vi "DAQ_Test.vi"() -> ()   [LabVIEW 2011]
uses:
  range_ni6009_TypDef.ctl
  OnOffTypeDef.ctl
panel:
  out "Array":variant[](array[variant])
  out "data 2":waveform(dbl)[](graph)
  in  "ChannelEnable":T1[](array[typedef])
  in  "range (V) 2":T2=enum."10"
  in  "Enable":bool
  in  "Channel (0.1.2.3)":string="0"
  in  "range (V)":T2=enum."10"
  in  "Range":T2[](array[typedef])
  out "Counter":i32
  out "OK":bool
  in  "timeout":dbl=1.0
  in  "Trigger":bool
  out "error out":errorcluster
  out "x-y":u32(graph)
  out "data":waveform(dbl)[](graph)
  in  "stop":bool
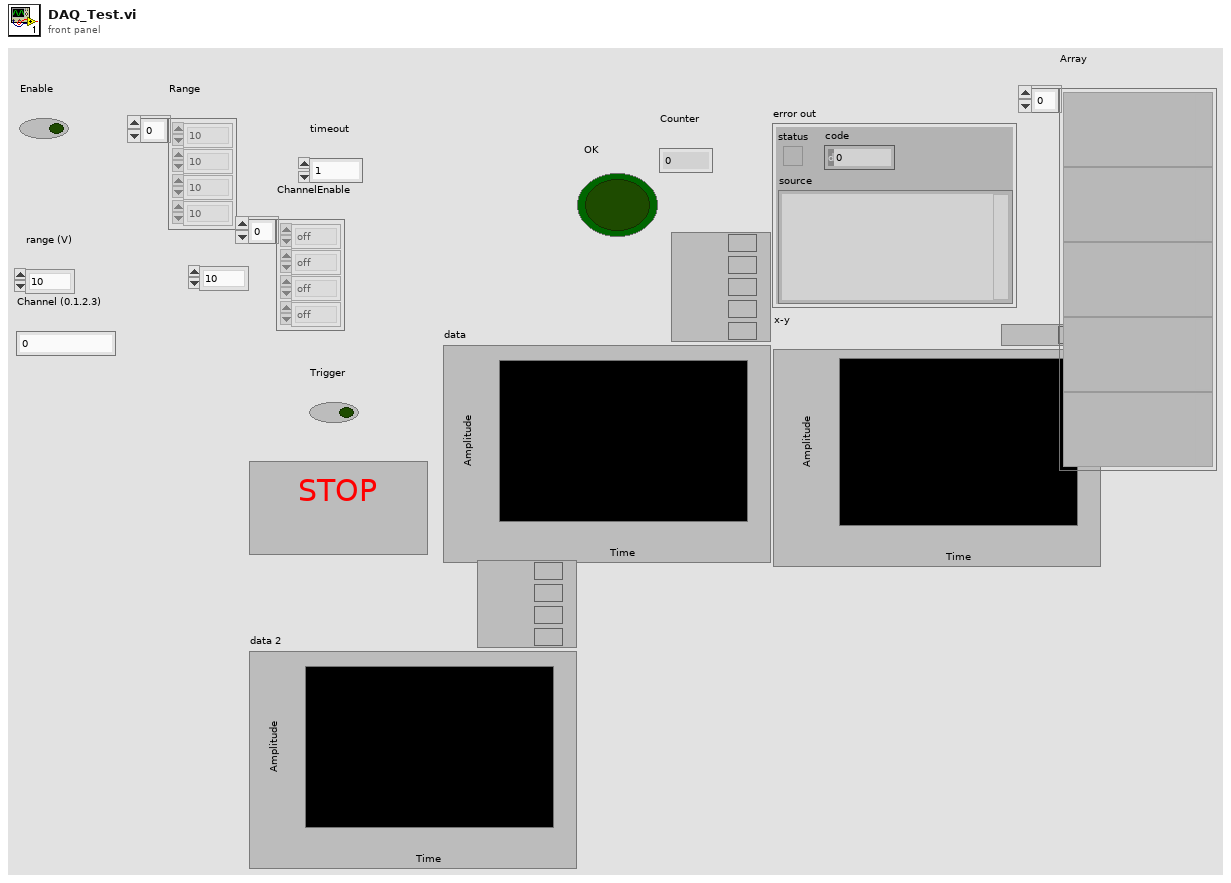
[diagram p1: front panel]
types:
  T1 = typedef "OnOffTypeDef.ctl" = enum16{"off", "on"}
  T2 = typedef "range_ni6009_TypDef.ctl" = enum16{"1", "2", "4", "5", "10"}
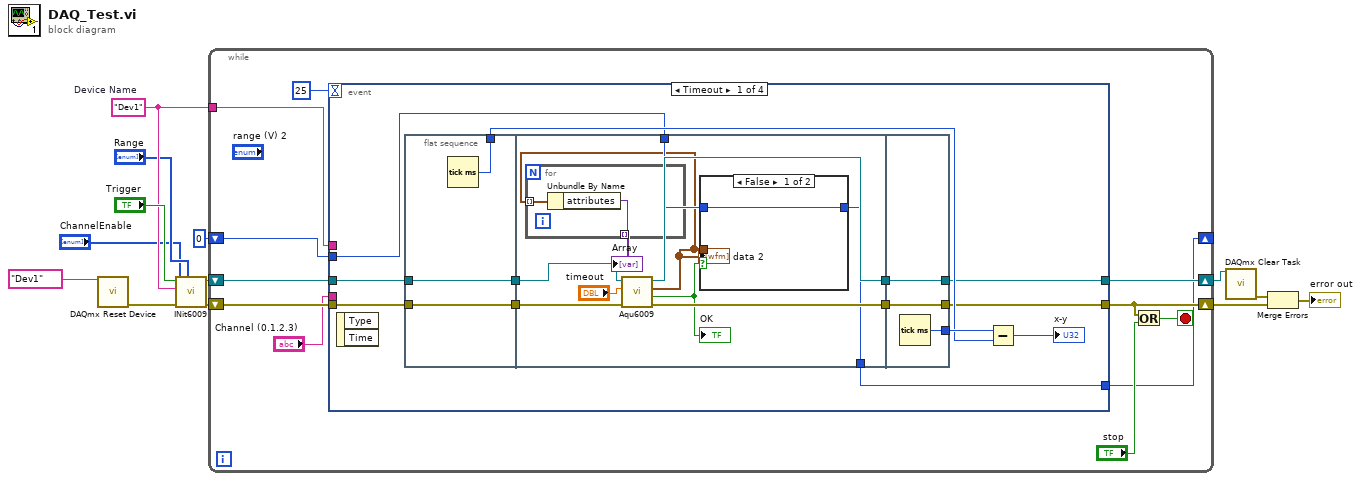
[diagram p0: block diagram]
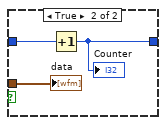
[diagram p2: hidden frame]
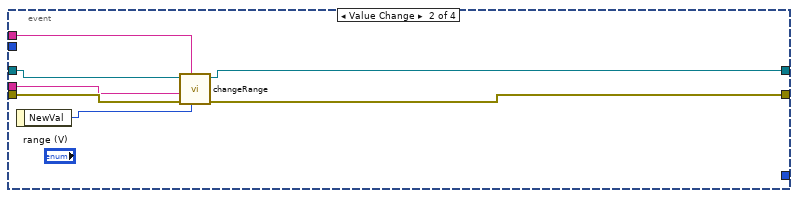
[diagram p3: hidden frame]
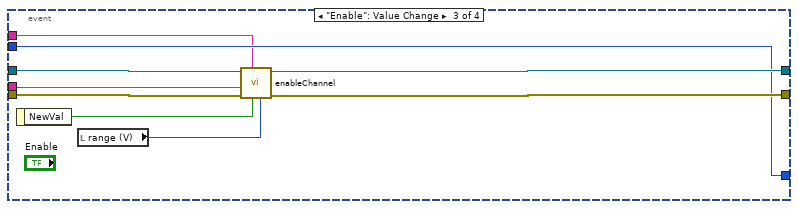
[diagram p4: hidden frame]
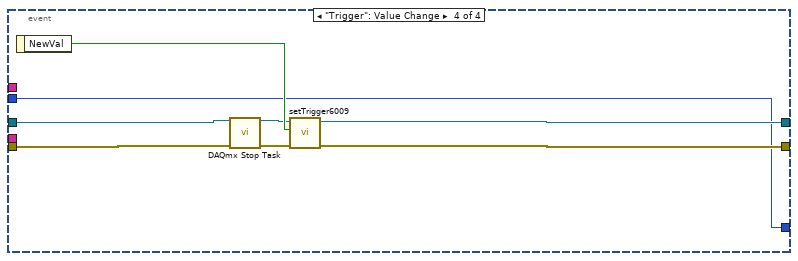
[diagram p5: hidden frame]
diagram:
  w4 = "Dev1"  # Device Name
  n1 = call "DAQmx Reset Device.vi"("device in"=tag "Dev1") -> ("error out"=w12:errorcluster)  [unwired: 14 in]
  n2 = call "INit6009.vi"("Range"="Range", "error in (no error)"=w12, "ChannelEnable"="ChannelEnable", "Device Name"=w4, "Trigger"="Trigger") -> ("error out"=w6:errorcluster, "Refnum out"=w7:refnum<k21>)  [unwired: 5 in]
  n3 = while {
    shift-right: [w19] -> w10
    shift-left: w6 -> [w20]
    shift-right: [w21] -> w8
    shift-left: w7 -> [w24]
    tunnel: w4 -> [w17]
    shift-right: [w15] -> _
    shift-left: 0 -> [w16]
    stop <- w22 stop-if-true
    n4 = event shown="[0] Timeout" {
      selector: _ -> [_ _ _ _]
      dyn-events: _ -> [_ _ _ _]
      timeout: 25 -> [_ _ _ _]
      tunnel: w24 -> [w25 w66 w72 w80]
      tunnel: [w31 w65 w74 w83] -> w21
      tunnel: w20 -> [w30 w64 w71 w78]
      tunnel: [w29 w63 w75 w82] -> w19
      tunnel: w17 -> [_ w62 w70 _]
      tunnel: w16 -> [w27 _ w73 w76]
      tunnel: [w26 _ w73 w76] -> w15
      tunnel: "Channel (0.1.2.3)" -> [_ w61 w69 _]
      event Timeout {
        n5 = event-data() -> ()  [unwired: 1 in, 2 out]
        n6 = flat-sequence {
          tunnel: w30 -> [w39]
          tunnel: w25 -> [w40]
          tunnel: [w40] -> w37
          tunnel: [w39] -> w36
          tunnel: [w38] -> w32
          tunnel: [w49] -> w35
          tunnel: w37 -> [w46]
          tunnel: w36 -> [w48]
          tunnel: [w47] -> w34
          tunnel: w27 -> [w44]
          tunnel: [w43] -> w26
          tunnel: [w59] -> w31
          tunnel: w35 -> [w59]
          tunnel: [w58] -> w33
          tunnel: [w57] -> w29
          tunnel: w34 -> [w57]
          frame #0 {
            n7 = Tick Count (ms)() -> (millisecond timer value=w38:u32)
          }
          frame #1 {
            n8 = call "Aqu6009.vi"("error in (no error)"=w48, "timeout"="timeout", "Refnum in"=w46) -> ("error out"=w47:errorcluster, "OK"=w45:bool, "data 2"=w42:waveform(dbl)[], "Refnum out"=w49:refnum<k21>)  [unwired: 5 in]
            "OK" <- w45
            "data 2" <- w42
            n9 = for {
              tunnel: w42 -> [w52] mode=indexing
              tunnel: [w51] -> w41 mode=indexing
              n10 = Unbundle By Name(w52) -> ("attributes"=w51:variant)
            }
            "Array" <- w41
            n11 = case shown="False" w45 {
              tunnel: w42 -> [_ w56]
              tunnel: w44 -> [w53 w55]
              tunnel: [w53 w54] -> w43
              frame False {
              }
              frame True {
                n12 = Increment(x=w55) -> (x+1=w54:i32)
                "Counter" <- w54
                "data" <- w56
              }
            }
          }
          frame #2 {
            n13 = Tick Count (ms)() -> (millisecond timer value=w58:u32)
          }
        }
        n14 = Subtract(x=w33, y=w32) -> (x-y=→"x-y":u32)
      }
      event Value Change {
        n15 = event-data() -> ("NewVal"=w60:T2)  [unwired: 1 in]
        n16 = call "changeRange.vi"("range (V)"=w60, "Device Name"=w62, "error in (no error)"=w64, "Channel (0.1.2.3)"=w61, "Refnum in"=w66) -> ("error out"=w63:errorcluster, "Refnum out"=w65:refnum<k21>)  [unwired: 5 in]
      }
      event "Enable": Value Change {
        n17 = event-data() -> ("NewVal"=w68:bool)  [unwired: 1 in]
        n18 = local read "range (V)"() -> (w67:T2)
        n19 = call "enableChannel.vi"("range (V)"=w67, "Enable"=w68, "Device Name"=w70, "error in (no error)"=w71, "Channel (0.1.2.3)"=w69, "Refnum in"=w72) -> ("error out"=w75:errorcluster, "Refnum out"=w74:refnum<k21>)  [unwired: 4 in]
      }
      event "Trigger": Value Change {
        n20 = event-data() -> ("NewVal"=w81:bool)  [unwired: 1 in]
        n21 = call "DAQmx Stop Task.vi"("task/channels in"=w80, "error in"=w78) -> ("task out"=w79:refnum<k21>, "error out"=w77:errorcluster)  [unwired: 12 in]
        n22 = call "setTrigger6009.vi"("error in (no error)"=w77, "Trigger"=w81, "Refnum in"=w79) -> ("error out"=w82:errorcluster, "Refnum out"=w83:refnum<k21>)  [unwired: 7 in]
      }
    }
    n23 = Or(x=w19, y="stop") -> (x .or. y?=w22:bool)
  }
  n24 = call "DAQmx Clear Task.vi"("task in"=w8) -> ("error out"=w11:errorcluster)  [unwired: 14 in]
  n25 = Merge Errors(w11, w10) -> (→"error out":errorcluster)
